vi "RFID_FTDI_Get-ID.vi"(8 "error in":errorcluster, 10 "Delay":u16=1200, 11 "COM RFID":refnum<visa-resource-name>="COM4") -> (0 "error out":errorcluster, 1 "Freq (Mhz)":dbl, 2 "RSSI":i32, 3 "Str EPC":string)   [LabVIEW 2018]
uses:
  utils/Return_t.ctl
  <vilib>/Instr/_visa.llb/VISA Configure Serial Port (Instr).vi
panel:
  out "FF?":bool
  out "Msg Length":u16
  out "Shift Data":u16
  out "Return":T1
  out "EPC Bytes":u8
  out "Read DATA Str":string
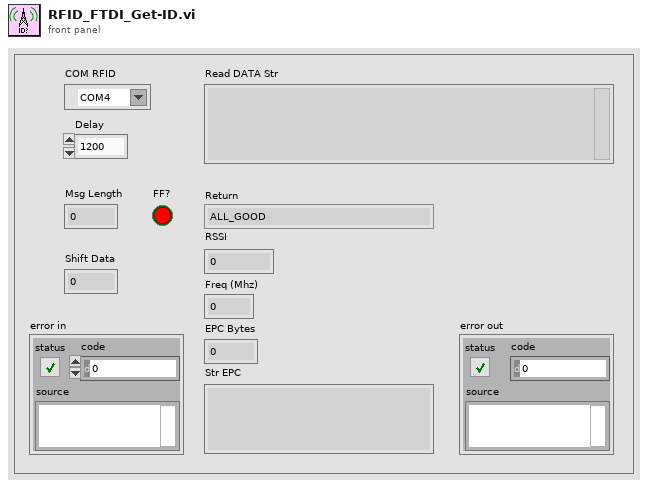
[diagram p1: front panel]
types:
  T1 = typedef "Return_t.ctl" = enum16{"ALL_GOOD", "ERROR_COMMAND_RESPONSE_TIMEOUT", "ERROR_CORRUPT_RESPONSE", "ERROR_WRONG_OPCODE_RESPONSE", "ERROR_UNKNOWN_OPCODE", "RESPONSE_IS_TEMPERATURE", "RESPONSE_IS_KEEPALIVE", "RESPONSE_IS_TEMPTHROTTLE", "RESPONSE_IS_TAGFOUND", "RESPONSE_IS_NOTAGFOUND", "RESPONSE_IS_UNKNOWN", "RESPONSE_SUCCESS", "RESPONSE_FAIL"}
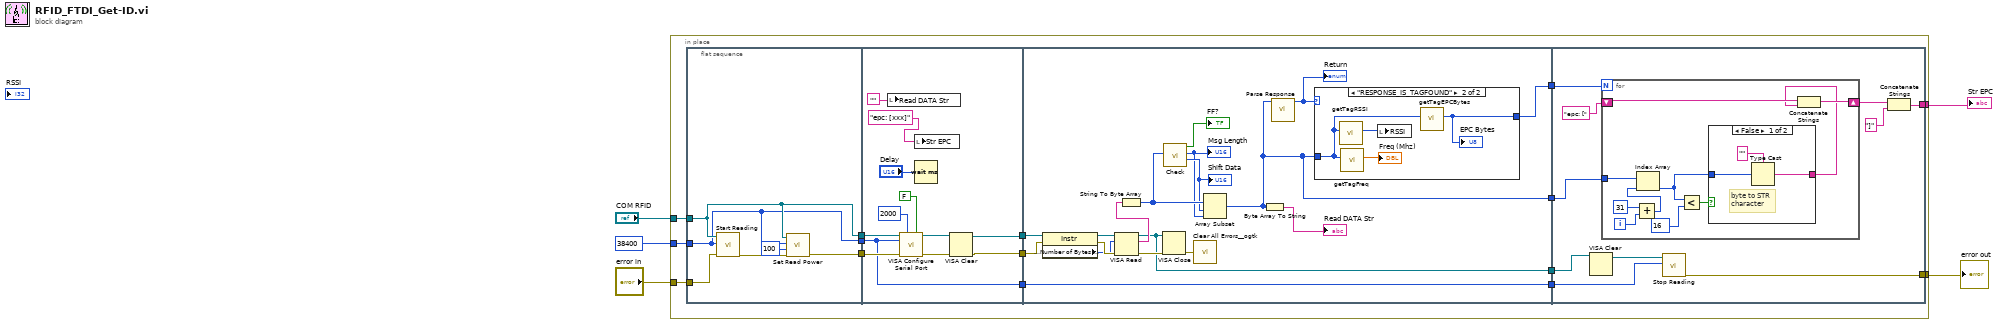
[diagram p0: block diagram]
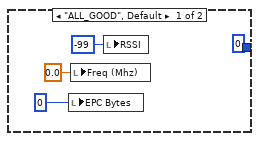
[diagram p2: hidden frame]
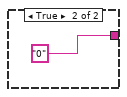
[diagram p3: hidden frame]
diagram:
  n1 = in-place {
    in-place-border: "error in" -> [w14]
    in-place-border: "COM RFID" -> [w13]
    in-place-border: [w12] -> w4
    in-place-border: [w11] -> w3
    in-place-border: 38400 -> [w10]
    n2 = flat-sequence {
      tunnel: w13 -> [w25]
      tunnel: w14 -> [w26]
      tunnel: w10 -> [w24]
      tunnel: [w24] -> w20
      tunnel: [w25] -> w19
      tunnel: [w22] -> w6
      tunnel: w20 -> [w27]
      tunnel: w19 -> [w37]
      tunnel: [w30] -> w18
      tunnel: [w29] -> w9
      tunnel: [w27] -> w8
      tunnel: w6 -> [w36]
      tunnel: [w44] -> w17
      tunnel: w18 -> [w56]
      tunnel: [w43] -> w16
      tunnel: [w42] -> w15
      tunnel: w9 -> [w55]
      tunnel: w8 -> [w39]
      tunnel: [w39] -> w7
      tunnel: w17 -> [w67]
      tunnel: [w74] -> w11
      tunnel: w16 -> [w73]
      tunnel: w15 -> [w70]
      tunnel: [w68] -> w12
      tunnel: w7 -> [w65]
      frame #0 {
        n3 = call "Start Reading.vi"("error in (no error)"=w26, "Baud Rate"=w24, "COM Port"=w25) -> ("error out"=w23:errorcluster)  [unwired: 6 in, 2 out]
        n4 = call "Set Read Power.vi"("error in (no error)"=w23, "Power"=u32 100, "Baud"=w24, "COM Port"=w25) -> ("error out"=w22:errorcluster)  [unwired: 5 in, 2 out]
      }
      frame #1 {
        n5 = local write "Read DATA Str"("") -> ()
        n6 = call-poly "VISA Configure Serial Port"("VISA resource name"=w37, "timeout (10sec)"=u32 2000, "Enable Termination\nChar (T)"=FALSE ("Enable Termination\nChar (T)"), "baud rate (9600)"=w27, "error in (no error)"=w36) -> ("VISA resource name out"=w31:refnum<visa-resource-name>, "error out"=w28:errorcluster)  [unwired: 9 in]
        n7 = local write "Str EPC"("epc: [xxx]") -> ()
        n8 = Wait (ms)(milliseconds to wait="Delay") -> ()  [unwired: 1 out]
        n9 = VISA Clear(VISA resource name=w31, error in (no error)=w28) -> (VISA resource name out=w30:refnum<visa-resource-name>, error out=w29:errorcluster)
      }
      frame #2 {
        n10 = property class="Instr"(reference=w56, error in=w55) -> (reference out=w52:refnum<visa-resource-name>, error out=w54:errorcluster, "Serial Settings:Number of Bytes at Serial Port"=w53:u32)
        n11 = VISA Read(VISA resource name=w52, byte count=w53, error in (no error)=w54) -> (VISA resource name out=w44:refnum<visa-resource-name>, read buffer=w45:string, error out=w47:errorcluster)  [unwired: 1 out]
        n12 = String To Byte Array(string=w45) -> (unsigned byte array=w51:u8[])
        n13 = VISA Close(VISA resource name=w44, error in (no error)=w47) -> (error out=w46:errorcluster)
        n14 = call "Check.vi"("Date"=w51) -> ("Shift Data"=w49:u16, "Msg Length"=w48:u16, "Result"=→"FF?":bool)  [unwired: 8 in]
        "Msg Length" <- w48
        "Shift Data" <- w49
        n15 = call <userlib>:"Clear All Errors__ogtk.vi"("Error In"=w46) -> ()  [unwired: 3 in, 1 out]
        n16 = Array Subset(array=w51, index=w49, length=w48) -> (w42:u8[])
        n17 = Byte Array To String(unsigned byte array=w42) -> (string=→"Read DATA Str":string)
        n18 = call "Parse Response.vi"("Data Array"=w42) -> ("Return"=w41:T1)  [unwired: 10 in]
        "Return" <- w41
        n19 = case shown="\"RESPONSE_IS_TAGFOUND\"" w41 {
          tunnel: w42 -> [_ w62]
          tunnel: [u8 0 ("EPC Bytes") w61] -> w43
          frame "ALL_GOOD", Default {
            n20 = local write "EPC Bytes"(u8 0 ("Butes Cnt")) -> ()
            n21 = local write "Freq (Mhz)"(0.0 ("Freq (Mhz)")) -> ()
            n22 = local write "RSSI"(-99 ("RSSI")) -> ()
          }
          frame "RESPONSE_IS_TAGFOUND" {
            n23 = call "getTagRSSI.vi"("Data Arry"=w62) -> ("RSSI"=w64:i32)  [unwired: 10 in]
            n24 = call "getTagFreq.vi"("Data Array"=w62) -> ("Freq"=→"Freq (Mhz)":dbl)  [unwired: 10 in]
            n25 = local write "RSSI"(w64) -> ()
            n26 = call "getTagEPCBytes.vi"("Data Arry"=w62) -> ("EPC Bytes"=w61:u8)  [unwired: 10 in]
            "EPC Bytes" <- w61
          }
        }
      }
      frame #3 {
        n27 = VISA Clear(VISA resource name=w67) -> (VISA resource name out=w66:refnum<visa-resource-name>)  [unwired: 1 in, 1 out]
        n28 = for {
          N: w73 -> [_]
          shift-right: [w83] -> w69
          shift-left: "epc: [" -> [w84]
          tunnel: w70 -> [w79]
          i -> [w82]
          n29 = Add(x=31, y=w82) -> (x+y=w80:i32)
          n30 = Index Array(array=w79, index=w80) -> (element=w76:u8)
          n31 = Less?(x=w76, y=u8 16) -> (x < y?=w77:bool)
          n32 = case shown="False" w77 {
            tunnel: w76 -> [w87 _]
            tunnel: [w86 "0"] -> w75
            frame False {
              # "byte to STR\ncharacter"
              n33 = Type Cast(type="", x=w87) -> (*(type *) &x=w86:string)
            }
            frame True {
            }
          }
          n34 = Concatenate Strings(w84, w75) -> (w83:string)
        }
        n35 = call "Stop Reading.vi"("Baud Rate"=w65, "COM Port"=w66) -> ("error out"=w74:errorcluster)  [unwired: 7 in, 2 out]
        n36 = Concatenate Strings(w69, "]" ("string")) -> (w68:string)
      }
    }
  }
  "Str EPC" <- w4
  "error out" <- w3
